vi "StartVideo.vi"() -> ()   [LabVIEW 2015]
uses:
  <vilib>/vision/Avi.llb/IMAQ AVI2 Codec Path.ctl
  <vilib>/vision/driver/IMAQdx.llb/IMAQdx Camera Control Mode.ctl
  <vilib>/userdefined/High Color/IMAQdx.ctl
  <vilib>/vision/Avi.llb/IMAQ AVI2 Refnum.ctl
  <vilib>/vision/driver/NI_Vision_Acquisition_Software.lvlib
panel:
  out "actual path":path
  out "Camera In":T1(plugin-control)
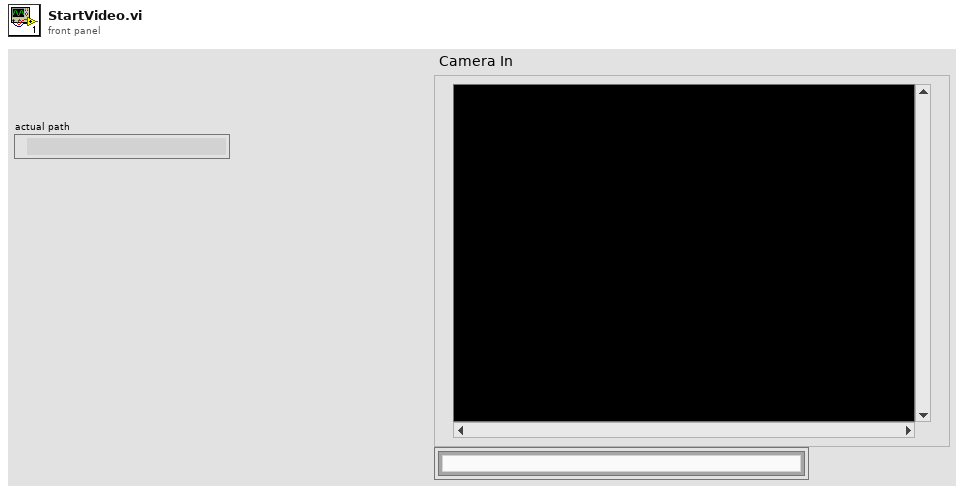
[diagram p1: front panel]
types:
  T1 = typedef "IMAQ Image.ctl" = refnum<image>
  T2 = typedef "IMAQ AVI2 Refnum.ctl" = refnum<k20>
  T3 = typedef "IMAQdx.ctl" = refnum<k21>
  T4 = typedef "NI_Vision_Acquisition_Software.lvlib/IMAQdx Camera Control Mode.ctl" = enum32{"Controller", "Listener"}
  T5 = typedef "IMAQ AVI2 Codec Path.ctl" = u32
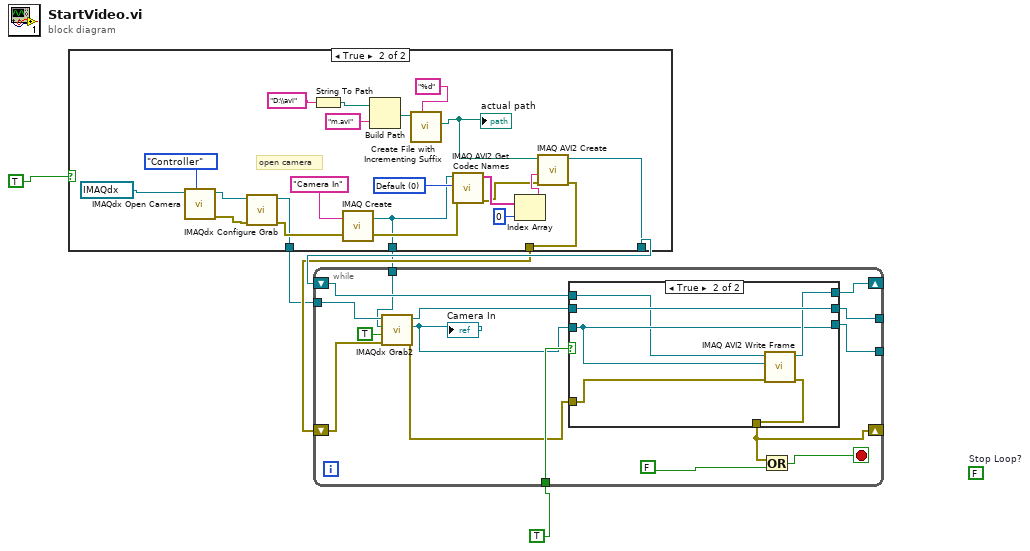
[diagram p0: block diagram]
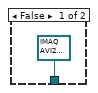
[diagram p2: hidden frame]
diagram:
  (unwired) FALSE  # Stop Loop?
  n1 = case shown="True" TRUE {
    tunnel: [T2 refnum ("AVI Refnum") w23] -> w6
    tunnel: [_ w15] -> w5
    tunnel: [_ w12] -> w4
    tunnel: [_ w11] -> w3
    frame False {
    }
    frame True {
      w27 = T5 0 items=["Default", "System", "Built in Vision"] ("Codec Source")
      # "open camera"
      n2 = call <vilib>:"IMAQdx Open Camera.vi"("Camera Control Mode"=IMAQdx_Camera_Control_Mode."Controller", "Session In"=T3 "cam1") -> ("error out"=w20:errorcluster, "Session Out"=w21:T3)  [unwired: 8 in]
      n3 = call <vilib>:"IMAQdx Configure Grab.vi"("error in"=w20, "Session In"=w21) -> ("error out"=w17:errorcluster, "Session Out"=w12:T3)  [unwired: 8 in]
      n4 = String To Path(string="D:\\avi") -> (path=w26:path)
      n5 = call "IMAQ Create"("Image Name"="Camera In", "error in (no error)"=w17) -> ("New Image"=w11:T1, "error out"=w13:errorcluster)  [unwired: 3 in]
      n6 = Build Path(base path=w26, name or relative path="m.avi") -> (appended path=w8:path)
      n7 = call "Create File with Incrementing Suffix.vi"("format string (\" (%d)\")"="%d" ("format string (\" (%d)\")"), "file path"=w8) -> ("actual path"=w10:path)  [unwired: 8 in, 1 out]
      "actual path" <- w10
      n8 = call "IMAQ AVI2 Get Codec Names"("error in (no error)"=w13, "Codec Source"=w27, "Image"=w11) -> ("error out"=w16:errorcluster, "Codec Names"=w29:string[])  [unwired: 7 in]
      n9 = Index Array(array=w29, index=0) -> (element=w28:string)
      n10 = call "IMAQ AVI2 Create"("error in (no error)"=w16, "Codec"=w28, "AVI Path"=w10) -> ("error out"=w15:errorcluster, "AVI Refnum"=w23:T2)  [unwired: 7 in]
    }
  }
  n11 = while {
    shift-right: [w33] -> _
    shift-left: w5 -> [w43]
    tunnel: w4 -> [w44]
    tunnel: [w40] -> _
    tunnel: [w38] -> _
    tunnel: TRUE -> [w42]
    shift-right: [w37] -> _
    shift-left: w6 -> [w35]
    tunnel: w3 -> [w32]
    stop <- w36 stop-if-true
    n12 = call <vilib>:"IMAQdx Grab2.vi"("error in"=w43, "Wait for Next Buffer? (Yes)"=TRUE, "Image In"=w32, "Session In"=w44) -> ("error out"=w34:errorcluster, "Image Out"=w39:T1, "Session Out"=w41:T3)  [unwired: 4 in, 1 out]
    "Camera In" <- w39
    n13 = case shown="True" w42 {
      tunnel: w41 -> [w48 w54]
      tunnel: [w48 w54] -> w40
      tunnel: w39 -> [w47 w52]
      tunnel: [w47 w52] -> w38
      tunnel: [w46 w53] -> w37
      tunnel: w35 -> [w46 w51]
      tunnel: w34 -> [w45 w50]
      tunnel: [w45 w49] -> w33
      frame False {
      }
      frame True {
        n14 = call "IMAQ AVI2 Write Frame"("error in (no error)"=w50, "Image"=w52, "AVI Refnum"=w51) -> ("error out"=w49:errorcluster, "AVI Refnum (duplicate)"=w53:T2)  [unwired: 6 in, 1 out]
      }
    }
    n15 = Or(x=w33, y=FALSE) -> (x .or. y?=w36:bool)
  }
